vi "RCMean.vi"(2 "Defect Flag array IN":i32[][](array[numeric]), 3 "data array in":dbl[](array[numeric]), 4 "No of strips":i32) -> (0 "standard deviation":dbl format="%.2f", 1 "mean":dbl format="%.2f")   [LabVIEW 2018]
uses:
  <vilib>/Analysis/NI_AALBase.lvlib
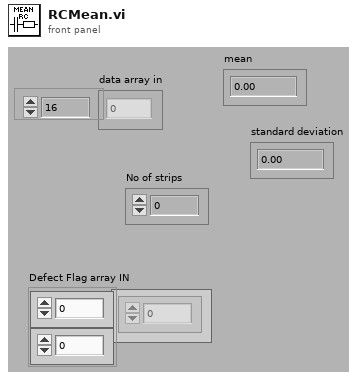
[diagram p1: front panel]
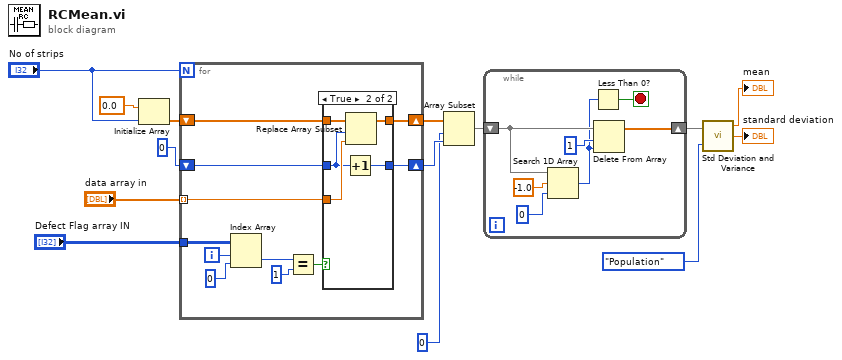
[diagram p0: block diagram]
diagram:
  n1 = Initialize Array(0.0, "No of strips") -> (w11:dbl[])
  n2 = for {
    N: "No of strips" -> [_]
    tunnel: "data array in" -> [w18] mode=indexing
    tunnel: "Defect Flag array IN" -> [w24]
    shift-right: [w15] -> w9
    shift-left: w11 -> [w19]
    shift-right: [w16] -> w8
    shift-left: 0 -> [w17]
    i -> [w21]
    n3 = Index Array(array=w24, index (row)=w21, index (col)=0) -> (element=w23:i32)
    n4 = Equal?(x=w23, y=1) -> (x = y?=w20:bool)
    n5 = case shown="True" w20 {
      tunnel: w19 -> [w27 w32]
      tunnel: w18 -> [_ w31]
      tunnel: w17 -> [w26 w28]
      tunnel: [w26 w30] -> w16
      tunnel: [w27 w29] -> w15
      frame False {
      }
      frame True {
        n6 = Increment(x=w28) -> (x+1=w30:i32)
        n7 = Replace Array Subset(array=w32, new element=w31, index=w28) -> (w29:dbl[])
      }
    }
  }
  n8 = Array Subset(array=w9, index=0, length=w8) -> (w2:dbl[])
  n9 = while {
    shift-right: [w36] -> w1
    shift-left: w2 -> [w35]
    stop <- w34 stop-if-true
    n10 = Search 1D Array(1D array=w35, element=-1.0, start index (0)=0) -> (index of element=w33:i32)
    n11 = Less Than 0?(x=w33) -> (x < 0?=w34:bool)
    n12 = Delete From Array(array=w35, length=1, index=w33) -> (array with subset deleted=w36:dbl[])  [unwired: 1 out]
  }
  n13 = call <vilib>:"Std Deviation and Variance.vi"("X"=w1, "Weighting (Sample)"=enum16{"Sample", "Population"}."Population") -> ("mean"=→"mean":dbl, "standard deviation"=→"standard deviation":dbl)  [unwired: 1 out]
